vi "setCornerWidget.vi"(8 "Error In":errorcluster, 10 "widget":refnum<class "QWidget.lvclass">, 11 "QAbstractScrollArea In":refnum<class "QAbstractScrollArea.lvclass">) -> (0 "Error Out":errorcluster, 3 "QAbstractScrollArea Out":refnum<class "QAbstractScrollArea.lvclass">)   [LabVIEW 2014, in "QAbstractScrollArea.lvclass"]
doc: "LabVIEW-specific documentation is not yet available. See <b>https://doc.qt.io/qt-5/qabstractscrollarea.html#setCornerWidget</b>"
uses:
  QAbstractScrollArea.lvclass
  QWidget/QWidget.lvclass
  LQ Core/LQIdentity/LQIdentity.lvclass/LQIdentity.ctl
  LQ Core/LQ Core.lvlib
  LQ Core/LQIdentity/LQIdentity.lvclass
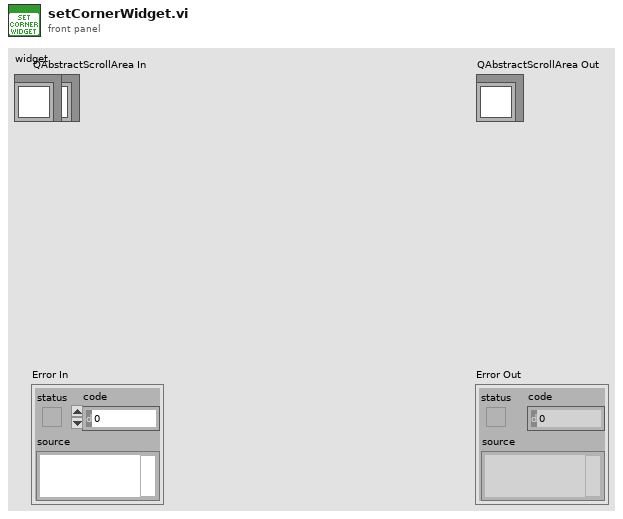
[diagram p1: front panel]
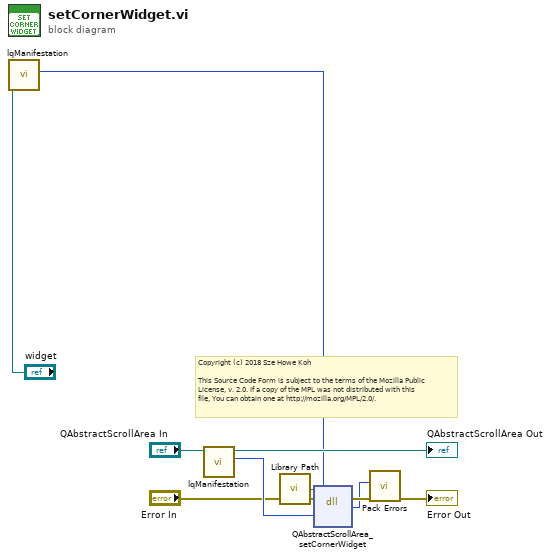
[diagram p0: block diagram]
diagram:
  # "Copyright (c) 2018 Sze Howe Koh\n\nThis Source Code Form is subject to the terms of the Mozilla Public\nLicense, v. 2.0. If a copy of the MPL was not distributed with this\nfile, You can obtain one at http://mozilla.org/MPL/2.0/."
  n1 = call "lqManifestation.vi"("LQIdentity in"="widget") -> ("Manifestation"=w1:u64)  [unwired: 9 in, 1 out]
  n2 = call "lqManifestation.vi"("LQIdentity in"="QAbstractScrollArea In") -> ("Manifestation"=w7:u64, "LQIdentity out"=→"QAbstractScrollArea Out":refnum<class "QAbstractScrollArea.lvclass">)  [unwired: 9 in]
  n3 = call "Library Path.vi"() -> ("Library Path"=w8:path)
  n4 = dll-call lib="?" fn="QAbstractScrollArea_setCornerWidget"(path in=w8, error in="Error In", "_instance"=w7, "widget"=w1) -> (error out=w5:errorcluster, w3:i32)  [unwired: 3 in, 1 out]
  n5 = call "Pack Errors.vi"("Error In"=w5, "Error Code"=w3) -> ("Error Out"=→"Error Out":errorcluster)  [unwired: 9 in]
